vi "Reactor Power.vi"(8 "Array":dbl[](array[numeric]), 9 "input cluster":T1, 10 "Shim Out":bool, 11 "Shim In":bool) -> (0 "SUR (DPM)":dbl, 1 "Reactor Power (%)":dbl, 2 "Reactor Power (W) out":dbl, 3 "Rod Height (cm) out":dbl, 4 "Change Reactivity":dbl)   [LabVIEW 2019]
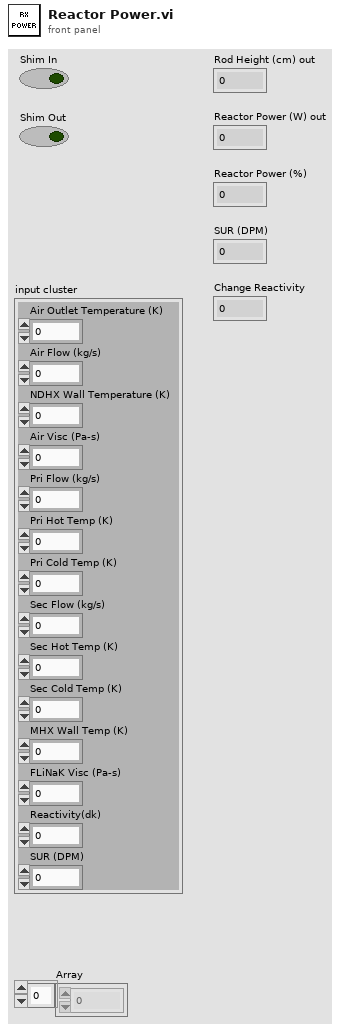
[diagram p1: front panel]
types:
  T1 = cluster{"Air Outlet Temperature (K)":dbl, "Air Flow (kg/s)":dbl, "NDHX Wall Temperature (K)":dbl, "Air Visc (Pa-s)":dbl, "Pri Flow (kg/s)":dbl, "Pri Hot Temp (K)":dbl, "Pri Cold Temp (K)":dbl, "Sec Flow (kg/s)":dbl, "Sec Hot Temp (K)":dbl, "Sec Cold Temp (K)":dbl, "MHX Wall Temp (K)":dbl, "FLiNaK Visc (Pa-s)":dbl, "Reactivity(dk)":dbl, "SUR (DPM)":dbl}
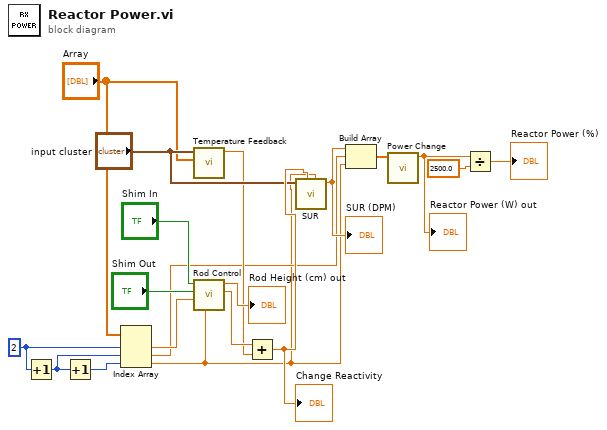
[diagram p0: block diagram]
diagram:
  w6 = 2 ("index")
  n1 = Increment(x=w6) -> (x+1=w5:i32)
  n2 = Increment(x=w5) -> (x+1=w4:i32)
  n3 = Index Array(array="Array", index #1=w6, index #2=w5, index #3=w4) -> (element #1=w3:dbl, element #2=w2:dbl, element #3=w1:dbl)
  n4 = call "Temperature Feedback.vi"("Temp Array"="Array", "input cluster"="input cluster") -> ("Change in Reactivity"=w14:dbl)  [unwired: 9 in]
  n5 = call "Rod Control.vi"("Time (s)"=w1, "Rod Height (cm) in"=w3, "Shim Out"="Shim Out", "Shim In"="Shim In") -> ("Change in Reactivity"=w17:dbl, "Rod Height (cm) out"=→"Rod Height (cm) out":dbl)  [unwired: 6 in]
  n6 = Add(x=w17, y=w14) -> (x+y=w16:dbl)
  "Change Reactivity" <- w16
  n7 = call "SUR.vi"("Time (s)"=w1, "Change Reactivity (dk)"=w16, "input cluster"="input cluster") -> ("SUR (DPM)"=w9:dbl)  [unwired: 8 in]
  "SUR (DPM)" <- w9
  n8 = Build Array(w9, w2, w1) -> (w8:dbl[])
  n9 = call "Power Change.vi"("Array"=w8) -> ("Reactor Power (W)"=w19:dbl)  [unwired: 10 in]
  "Reactor Power (W) out" <- w19
  n10 = Divide(x=w19, y=2500.0) -> (x/y=→"Reactor Power (%)":dbl)
